vi "Send.vi"(8 "error in":errorcluster, 11 "Block Upload End Transfer in":refnum<class "Block Upload End Transfer.lvclass">) -> (0 "error out":errorcluster, 3 "Block Upload End Transfer out":refnum<class "Block Upload End Transfer.lvclass">)   [LabVIEW 2020, in "CANopen.lvlib" / "SDO Manager.lvlib" / "Block Upload End Transfer.lvclass"]
uses:
  Block Upload End Transfer.lvclass
  HAL/Source/Interfaces/ICommunicate/ICommunicate.lvclass
  CANopen Message/CANopen Message.lvclass
  Typedefs/Function Code.ctl
  CANopen.lvlib
  SDO Transfer/SDO Transfer.lvclass
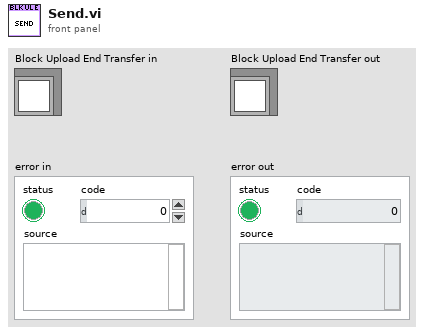
[diagram p1: front panel]
types:
  T1 = typedef "CANopen.lvlib/Function Code.ctl" = u8
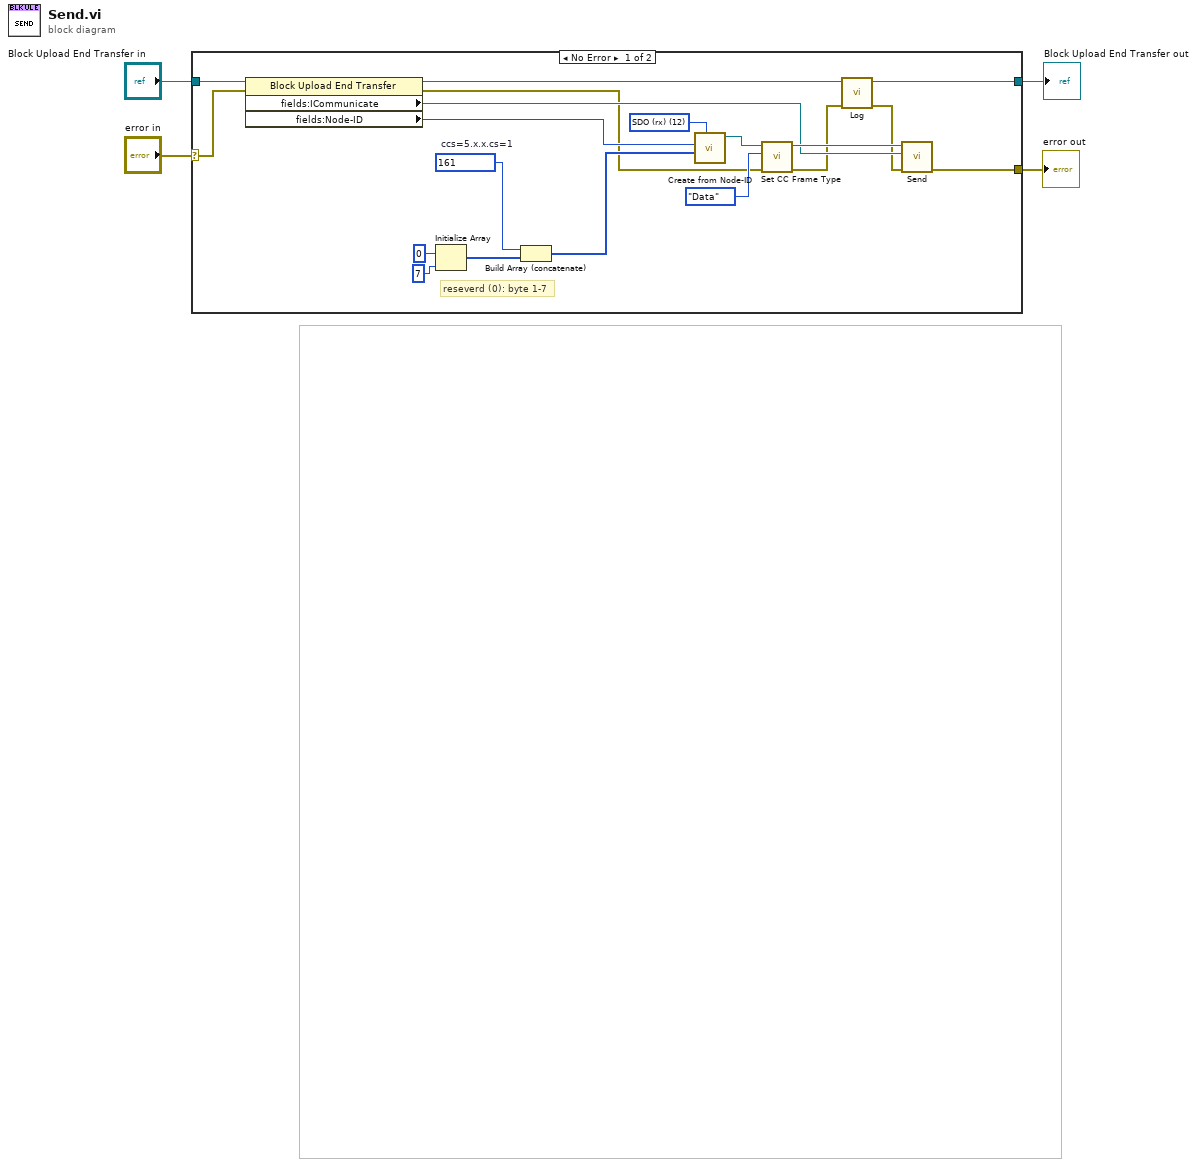
[diagram p0: block diagram]
diagram:
  n1 = case shown="No Error" "error in" {
    selector: "error in" -> [w23 w24]
    tunnel: "Block Upload End Transfer in" -> [w22 w25]
    tunnel: [w10 w25] -> w1
    tunnel: [w9 w24] -> w2
    frame No Error {
      w17 = T1 12 items=["NMT"=0, "EMCY/SYNC"=1, "TIME"=2, "PDO1 (tx)"=3, "PDO1 (rx)"=4, "PDO2 (tx)"=5, "PDO2 (rx)"=6, "PDO3 (tx)"=7, "PDO3 (rx)"=8, "PDO4 (tx)"=9, "PDO4 (rx)"=10, "SDO (tx)"=11, "SDO (rx)"=12, "NMT error control"=14] ("Function Code")
      w20 = u8 161  # ccs=5.x.x.cs=1
      # "reseverd (0): byte 1-7"
      n2 = property class="Block Upload End Transfer"(reference=w22, error in=w23) -> (reference out=w11:refnum<class "Block Upload End Transfer.lvclass">, error out=w8:errorcluster, "fields:ICommunicate"=w12:refnum<class "ICommunicate.lvclass">, "fields:Node-ID"=w21:u8)
      n3 = Initialize Array(u8 0, 7 ("y")) -> (w5:u8[])
      n4 = Build Array (concatenate)(w20, w5) -> (w18:u8[])
      n5 = call "Create from Node-ID.vi"("Function Code"=w17, "Data"=w18, "Node-ID"=w21) -> ("CANopen Message"=w16:refnum<class "CANopen Message.lvclass">)  [unwired: 8 in]
      n6 = call "Set CC Frame Type.vi"("error in"=w8, "CC Frame Type"=enum8{"Data", "Remote", "Error", "Overload"}."Data", "CANopen Message in"=w16) -> ("error out"=w7:errorcluster, "CANopen Message out"=w15:refnum<class "CANopen Message.lvclass">)  [unwired: 7 in]
      n7 = call "Log.vi"("error in"=w7, "SDO Transfer in"=w11) -> ("error out"=w6:errorcluster, "SDO Transfer out"=w10:refnum<class "Block Upload End Transfer.lvclass">)  [unwired: 8 in]
      n8 = call "Send.vi"("error in"=w6, "ICommunicate"=w12, "CANopen Message in"=w15) -> ("error out"=w9:errorcluster)  [unwired: 7 in, 1 out]
    }
    frame Error {
    }
  }
  "Block Upload End Transfer out" <- w1
  "error out" <- w2
